vi "Auton - Far Gear.vi"(10 "Alliance":T2, 11 "Auton States":T1=enum."Reset Encoders") -> ()   [LabVIEW 2016]
uses:
  <vilib>/Rock Robotics/WPI/DriverStation/WPI_DriverStationAllianceInfo.ctl
  Auton - Far Gear States.ctl
panel:
  in  "Turn Adjust Blue":dbl=294.0
  in  "Turn Adjust Red":dbl=65.0
  out "Current State":T1
  in  "Mount Peg Distance SP":dbl=17.0
  in  "Back Away SP":dbl
  in  "Drive Distance to Airship SP":dbl=42.0
  in  "Red - Face Airship Gyro SP":dbl=56.0
  in  "Blue - Face Airship Gyro SP":dbl=304.0
  in  "Drive Forward SP":dbl=72.0
  # "76"
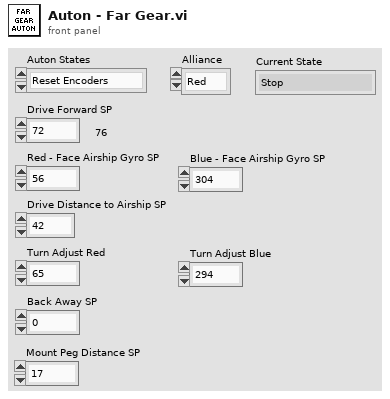
[diagram p1: front panel]
types:
  T1 = typedef "Auton - Far Gear States.ctl" = enum16{"Stop", "Reset Encoders", "Drive Forward", "Face Airship Gyro", "Reset Encoders Again", "Drive Forward to Peg", "Turn to Mount Peg", "Reset Encoders Again Again", "Mount Peg", "Eject Gear", "Back Away"}
  T2 = typedef "WPI_DriverStationAllianceInfo.ctl" = enum16{"Red", "Blue", "Invalid"}
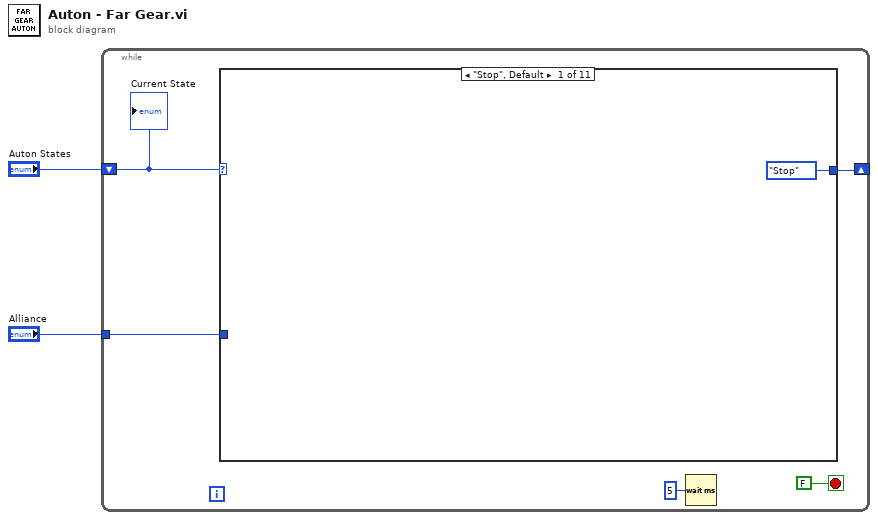
[diagram p0: block diagram]
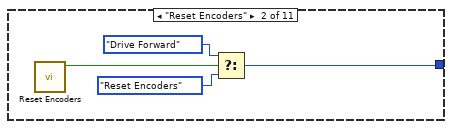
[diagram p2: hidden frame]
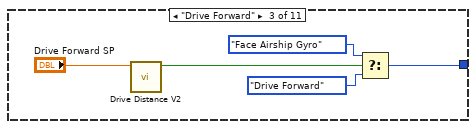
[diagram p3: hidden frame]
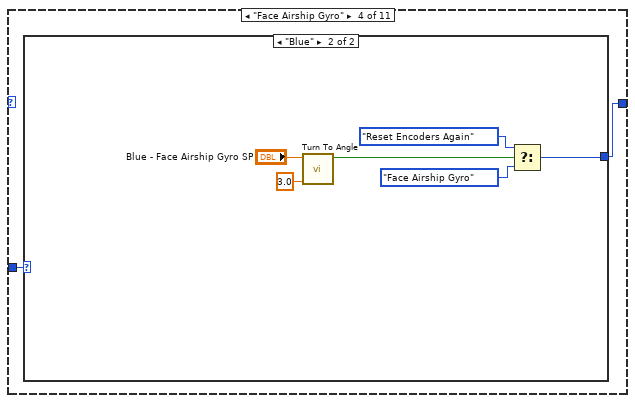
[diagram p4: hidden frame]
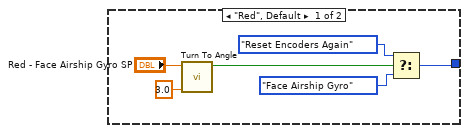
[diagram p5: hidden frame]
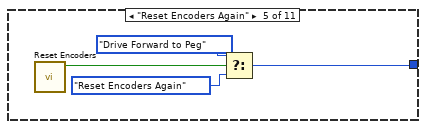
[diagram p6: hidden frame]
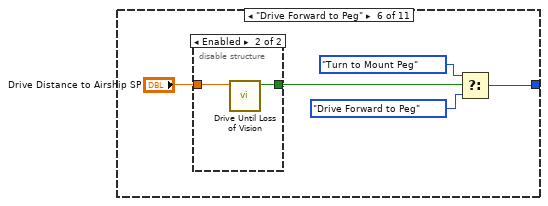
[diagram p7: hidden frame]
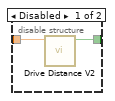
[diagram p8: hidden frame]
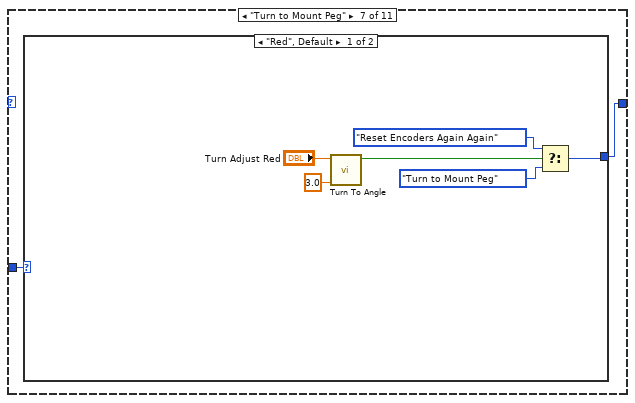
[diagram p9: hidden frame]
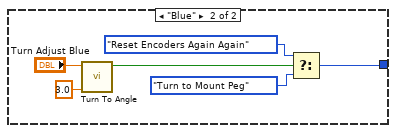
[diagram p10: hidden frame]
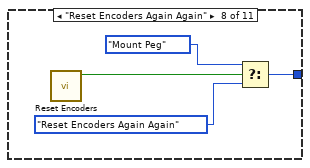
[diagram p11: hidden frame]
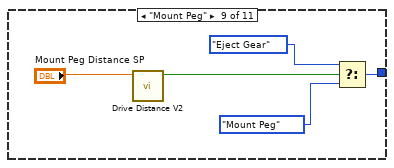
[diagram p12: hidden frame]
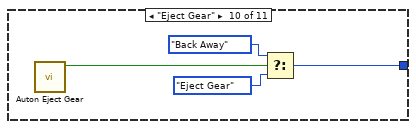
[diagram p13: hidden frame]
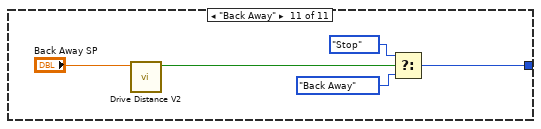
[diagram p14: hidden frame]
diagram:
  n1 = while {
    shift-right: [w7] -> _
    shift-left: "Auton States" -> [w3]
    tunnel: "Alliance" -> [w6]
    stop <- FALSE stop-if-true
    n2 = case shown="\"Stop\", Default" w3 {
      tunnel: [Auton_-_Far_Gear_States."Stop" ("Auton States") w9 w15 w18 w32 w38 w45 w60 w64 w69 w74] -> w7
      tunnel: w6 -> [_ _ _ w19 _ _ w46 _ _ _ _]
      frame "Stop", Default {
      }
      frame "Reset Encoders" {
        n3 = call "Reset Encoders.vi"() -> ("Done?"=w12:bool)  [unwired: 11 in]
        n4 = Select(t=Auton_-_Far_Gear_States."Drive Forward" ("Auton States"), s=w12, f=Auton_-_Far_Gear_States."Reset Encoders" ("Auton States")) -> (s? t:f=w9:T1)
      }
      frame "Drive Forward" {
        n5 = call "Drive Distance V2.vi"("Distance Set Point"="Drive Forward SP") -> ("Done?"=w14:bool)  [unwired: 10 in]
        n6 = Select(t=Auton_-_Far_Gear_States."Face Airship Gyro" ("Auton States"), s=w14, f=Auton_-_Far_Gear_States."Drive Forward" ("Auton States")) -> (s? t:f=w15:T1)
      }
      frame "Face Airship Gyro" {
        n7 = case shown="\"Blue\"" w19 {
          tunnel: [w21 w29] -> w18
          frame "Red", Default {
            n8 = call "Turn To Angle.vi"("Turn Angle Tolerance"=3.0, "Setpoint"="Red - Face Airship Gyro SP") -> ("Done?"=w24:bool)  [unwired: 9 in]
            n9 = Select(t=Auton_-_Far_Gear_States."Reset Encoders Again" ("Auton States"), s=w24, f=Auton_-_Far_Gear_States."Face Airship Gyro" ("Auton States")) -> (s? t:f=w21:T1)
          }
          frame "Blue" {
            n10 = call "Turn To Angle.vi"("Turn Angle Tolerance"=3.0, "Setpoint"="Blue - Face Airship Gyro SP") -> ("Done?"=w28:bool)  [unwired: 9 in]
            n11 = Select(t=Auton_-_Far_Gear_States."Reset Encoders Again" ("Auton States"), s=w28, f=Auton_-_Far_Gear_States."Face Airship Gyro" ("Auton States")) -> (s? t:f=w29:T1)
          }
        }
      }
      frame "Reset Encoders Again" {
        n12 = call "Reset Encoders.vi"() -> ("Done?"=w33:bool)  [unwired: 11 in]
        n13 = Select(t=Auton_-_Far_Gear_States."Drive Forward to Peg" ("Auton States"), s=w33, f=Auton_-_Far_Gear_States."Reset Encoders Again" ("Auton States")) -> (s? t:f=w32:T1)
      }
      frame "Drive Forward to Peg" {
        n14 = disable-structure shown="Enabled" {
          disable-tunnel: "Drive Distance to Airship SP" -> [w42 w44]
          disable-tunnel: [w41 w43] -> w36
          frame Disabled {
            n15 = call "Drive Distance V2.vi"("Distance Set Point"=w42) -> ("Done?"=w41:bool)  [unwired: 10 in]
          }
          frame Enabled {
            n16 = call "Drive Until Loss of Vision.vi"("Distance Setpoint"=w44) -> ("ready to approach"=w43:bool)  [unwired: 10 in]
          }
        }
        n17 = Select(t=Auton_-_Far_Gear_States."Turn to Mount Peg" ("Auton States"), s=w36, f=Auton_-_Far_Gear_States."Drive Forward to Peg" ("Auton States")) -> (s? t:f=w38:T1)
      }
      frame "Turn to Mount Peg" {
        n18 = case shown="\"Red\", Default" w46 {
          tunnel: [w48 w56] -> w45
          frame "Red", Default {
            n19 = call "Turn To Angle.vi"("Turn Angle Tolerance"=3.0, "Setpoint"="Turn Adjust Red") -> ("Done?"=w51:bool)  [unwired: 9 in]
            n20 = Select(t=Auton_-_Far_Gear_States."Reset Encoders Again Again" ("Auton States"), s=w51, f=Auton_-_Far_Gear_States."Turn to Mount Peg" ("Auton States")) -> (s? t:f=w48:T1)
          }
          frame "Blue" {
            n21 = call "Turn To Angle.vi"("Turn Angle Tolerance"=3.0, "Setpoint"="Turn Adjust Blue") -> ("Done?"=w55:bool)  [unwired: 9 in]
            n22 = Select(t=Auton_-_Far_Gear_States."Reset Encoders Again Again" ("Auton States"), s=w55, f=Auton_-_Far_Gear_States."Turn to Mount Peg" ("Auton States")) -> (s? t:f=w56:T1)
          }
        }
      }
      frame "Reset Encoders Again Again" {
        n23 = call "Reset Encoders.vi"() -> ("Done?"=w59:bool)  [unwired: 11 in]
        n24 = Select(t=Auton_-_Far_Gear_States."Mount Peg" ("Auton States"), s=w59, f=Auton_-_Far_Gear_States."Reset Encoders Again Again" ("Auton States")) -> (s? t:f=w60:T1)
      }
      frame "Mount Peg" {
        n25 = call "Drive Distance V2.vi"("Distance Set Point"="Mount Peg Distance SP") -> ("Done?"=w63:bool)  [unwired: 10 in]
        n26 = Select(t=Auton_-_Far_Gear_States."Eject Gear" ("Auton States"), s=w63, f=Auton_-_Far_Gear_States."Mount Peg" ("Auton States")) -> (s? t:f=w64:T1)
      }
      frame "Eject Gear" {
        n27 = call "Auton Eject Gear.vi"() -> ("Done?"=w68:bool)  [unwired: 11 in]
        n28 = Select(t=Auton_-_Far_Gear_States."Back Away" ("Auton States"), s=w68, f=Auton_-_Far_Gear_States."Eject Gear" ("Auton States")) -> (s? t:f=w69:T1)
      }
      frame "Back Away" {
        n29 = call "Drive Distance V2.vi"("Distance Set Point"="Back Away SP") -> ("Done?"=w73:bool)  [unwired: 10 in]
        n30 = Select(t=Auton_-_Far_Gear_States."Stop" ("Auton States"), s=w73, f=Auton_-_Far_Gear_States."Back Away" ("Auton States")) -> (s? t:f=w74:T1)
      }
    }
    n31 = Wait (ms)(milliseconds to wait=u32 5) -> ()  [unwired: 1 out]
    "Current State" <- w3
  }
